vi "MeasLeakRate01.vi"() -> ()   [LabVIEW 2011]
panel:
  out "leak rate (torr/min)":dbl
  out "S20":dbl
  out "S11":dbl
  out "S10":dbl
  out "S01":dbl
  out "S00":dbl
  out "A11":dbl[](array[numeric])
  out "P":dbl
  in  "first":bool=TRUE
  out "A20":dbl[](array[numeric])
  out "A10":dbl[](array[numeric])
  out "A01":dbl[](array[numeric])
  out "A00":dbl[](array[numeric])
  in  "interval (s)":dbl
  in  "stop":bool
  out "P(Torr)":string
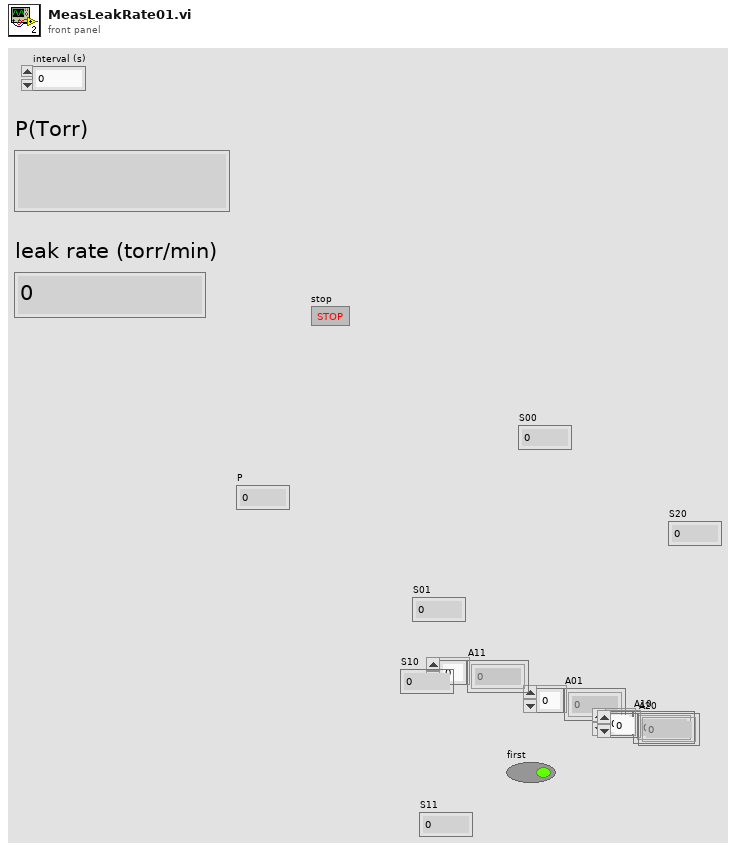
[diagram p1: front panel]
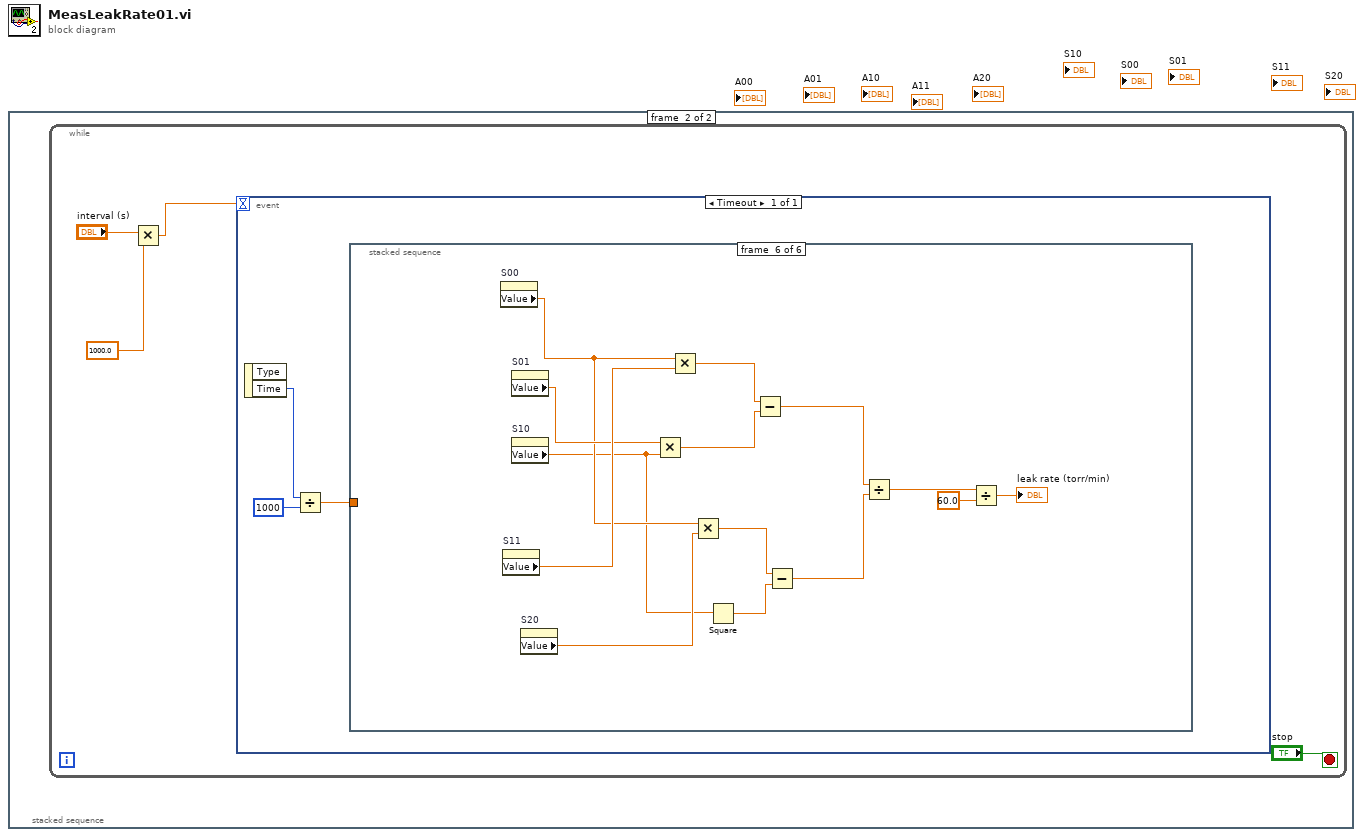
[diagram p0: block diagram]
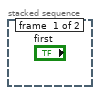
[diagram p2: hidden frame]
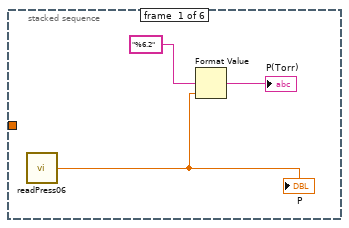
[diagram p3: hidden frame]
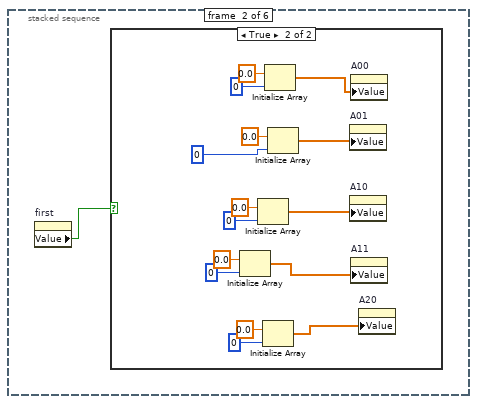
[diagram p4: hidden frame]
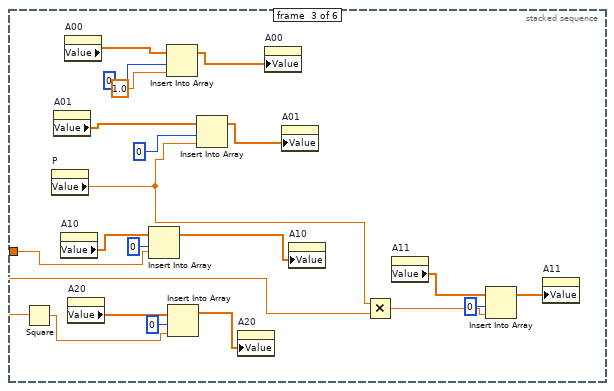
[diagram p6: hidden frame]
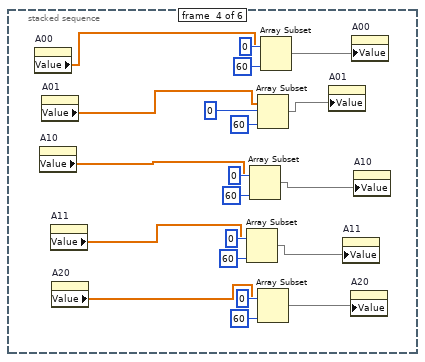
[diagram p7: hidden frame]
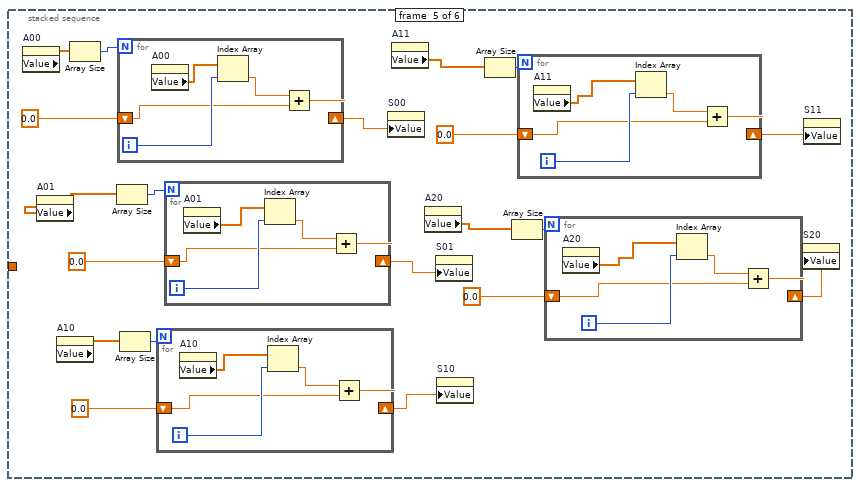
[diagram p8: hidden frame]
diagram:
  n1 = stacked-sequence {
    frame #0 {
    }
    frame #1 {
      n2 = while {
        stop <- "stop" stop-if-true
        n3 = Multiply(x="interval (s)", y=1000.0) -> (x*y=w2:dbl)
        n4 = event shown="[0] Timeout" {
          selector: _ -> [_]
          dyn-events: _ -> [_]
          timeout: w2 -> [_]
          event Timeout {
            n5 = event-data() -> ("Time"=w7:u32)  [unwired: 1 in, 1 out]
            n6 = Divide(x=w7, y=u32 1000) -> (x/y=w5:dbl)
            n7 = stacked-sequence {
              tunnel: w5 -> [_ _ w36 _ _ _]
              frame #0 {
                n8 = call "readPress06.vi"() -> ("P"=w9:dbl)
                "P" <- w9
                n9 = Format Value(format string="%6.2", value (0)=w9) -> (output string=→"P(Torr)":string)  [unwired: 1 in]
              }
              frame #1 {
                n10 = property on="first" class="Bool (strict)"() -> ("Value"=w11:bool)  [unwired: 2 in, 2 out]
                n11 = case shown="True" w11 {
                  frame False {
                  }
                  frame True {
                    n12 = Initialize Array(0.0 ("element"), 0 ("dimension size")) -> (w14:dbl[])
                    n13 = Initialize Array(0.0 ("element"), 0 ("dimension size")) -> (w15:dbl[])
                    n14 = Initialize Array(0.0 ("element"), 0 ("dimension size")) -> (w13:dbl[])
                    n15 = Initialize Array(0.0 ("element"), 0 ("dimension size")) -> (w12:dbl[])
                    n16 = Initialize Array(0.0 ("element"), 0 ("dimension size")) -> (w16:dbl[])
                    n17 = property on="A01" class="Arr (strict)"("Value"=w16) -> ()  [unwired: 2 in, 2 out]
                    n18 = property on="A10" class="Arr (strict)"("Value"=w15) -> ()  [unwired: 2 in, 2 out]
                    n19 = property on="A00" class="Arr (strict)"("Value"=w12) -> ()  [unwired: 2 in, 2 out]
                    n20 = property on="A11" class="Arr (strict)"("Value"=w14) -> ()  [unwired: 2 in, 2 out]
                    n21 = property on="A20" class="Arr (strict)"("Value"=w13) -> ()  [unwired: 2 in, 2 out]
                  }
                }
              }
              frame #2 {
                n22 = Square(x=w36) -> (x^2=w37:dbl)
                n23 = property on="P" class="DigNum (strict)"() -> ("Value"=w35:dbl)  [unwired: 2 in, 2 out]
                n24 = property on="A01" class="Arr (strict)"() -> ("Value"=w42:dbl[])  [unwired: 2 in, 2 out]
                n25 = property on="A10" class="Arr (strict)"() -> ("Value"=w41:dbl[])  [unwired: 2 in, 2 out]
                n26 = property on="A00" class="Arr (strict)"() -> ("Value"=w44:dbl[])  [unwired: 2 in, 2 out]
                n27 = property on="A20" class="Arr (strict)"() -> ("Value"=w39:dbl[])  [unwired: 2 in, 2 out]
                n28 = Insert Into Array(array=w41, index=0, new element=w36) -> (w29:dbl[])
                n29 = Insert Into Array(array=w44, index=0, new element=1.0 ("new element/subarray")) -> (w31:dbl[])
                n30 = Insert Into Array(array=w39, index=0, new element=w37) -> (w30:dbl[])
                n31 = Insert Into Array(array=w42, index=0, new element=w35) -> (w27:dbl[])
                n32 = property on="A20" class="Arr (strict)"("Value"=w30) -> ()  [unwired: 2 in, 2 out]
                n33 = property on="A00" class="Arr (strict)"("Value"=w31) -> ()  [unwired: 2 in, 2 out]
                n34 = property on="A01" class="Arr (strict)"("Value"=w27) -> ()  [unwired: 2 in, 2 out]
                n35 = property on="A10" class="Arr (strict)"("Value"=w29) -> ()  [unwired: 2 in, 2 out]
                n36 = Multiply(x=w35, y=w36) -> (x*y=w33:dbl)
                n37 = property on="A11" class="Arr (strict)"() -> ("Value"=w34:dbl[])  [unwired: 2 in, 2 out]
                n38 = Insert Into Array(array=w34, index=0, new element=w33) -> (w28:dbl[])
                n39 = property on="A11" class="Arr (strict)"("Value"=w28) -> ()  [unwired: 2 in, 2 out]
              }
              frame #3 {
                n40 = property on="A00" class="Arr (strict)"() -> ("Value"=w61:dbl[])  [unwired: 2 in, 2 out]
                n41 = property on="A10" class="Arr (strict)"() -> ("Value"=w52:dbl[])  [unwired: 2 in, 2 out]
                n42 = property on="A01" class="Arr (strict)"() -> ("Value"=w53:dbl[])  [unwired: 2 in, 2 out]
                n43 = property on="A11" class="Arr (strict)"() -> ("Value"=w51:dbl[])  [unwired: 2 in, 2 out]
                n44 = property on="A20" class="Arr (strict)"() -> ("Value"=w64:dbl[])  [unwired: 2 in, 2 out]
                n45 = Array Subset(array=w51, index=0, length=60) -> (w48:dbl[])
                n46 = Array Subset(array=w52, index=0, length=60) -> (w49:dbl[])
                n47 = Array Subset(array=w53, index=0, length=60) -> (w50:dbl[])
                n48 = Array Subset(array=w64, index=0, length=60) -> (w47:dbl[])
                n49 = Array Subset(array=w61, index=0, length=60) -> (w60:dbl[])
                n50 = property on="A01" class="Arr (strict)"("Value"=w50) -> ()  [unwired: 2 in, 2 out]
                n51 = property on="A11" class="Arr (strict)"("Value"=w48) -> ()  [unwired: 2 in, 2 out]
                n52 = property on="A20" class="Arr (strict)"("Value"=w47) -> ()  [unwired: 2 in, 2 out]
                n53 = property on="A00" class="Arr (strict)"("Value"=w60) -> ()  [unwired: 2 in, 2 out]
                n54 = property on="A10" class="Arr (strict)"("Value"=w49) -> ()  [unwired: 2 in, 2 out]
              }
              frame #4 {
                n55 = property on="A00" class="Arr (strict)"() -> ("Value"=w85:dbl[])  [unwired: 2 in, 2 out]
                n56 = property on="A01" class="Arr (strict)"() -> ("Value"=w81:dbl[])  [unwired: 2 in, 2 out]
                n57 = property on="A10" class="Arr (strict)"() -> ("Value"=w78:dbl[])  [unwired: 2 in, 2 out]
                n58 = Array Size(array=w85) -> (size(s)=w86:i32)
                n59 = Array Size(array=w81) -> (size(s)=w83:i32)
                n60 = for {
                  N: w86 -> [_]
                  shift-right: [w107] -> w71
                  shift-left: 0.0 -> [w108]
                  i -> [w110]
                  n61 = property on="A00" class="Arr (strict)"() -> ("Value"=w111:dbl[])  [unwired: 2 in, 2 out]
                  n62 = Index Array(array=w111, index=w110) -> (element=w109:dbl)
                  n63 = Add(x=w109, y=w108) -> (x+y=w107:dbl)
                }
                n64 = Array Size(array=w78) -> (size(s)=w80:i32)
                n65 = for {
                  N: w80 -> [_]
                  shift-right: [w98] -> w70
                  shift-left: 0.0 -> [w99]
                  i -> [w101]
                  n66 = property on="A10" class="Arr (strict)"() -> ("Value"=w97:dbl[])  [unwired: 2 in, 2 out]
                  n67 = Index Array(array=w97, index=w101) -> (element=w100:dbl)
                  n68 = Add(x=w100, y=w99) -> (x+y=w98:dbl)
                }
                n69 = for {
                  N: w83 -> [_]
                  shift-right: [w103] -> w69
                  shift-left: 0.0 -> [w104]
                  i -> [w106]
                  n70 = property on="A01" class="Arr (strict)"() -> ("Value"=w102:dbl[])  [unwired: 2 in, 2 out]
                  n71 = Index Array(array=w102, index=w106) -> (element=w105:dbl)
                  n72 = Add(x=w105, y=w104) -> (x+y=w103:dbl)
                }
                n73 = property on="S00" class="DigNum (strict)"("Value"=w71) -> ()  [unwired: 2 in, 2 out]
                n74 = property on="A11" class="Arr (strict)"() -> ("Value"=w75:dbl[])  [unwired: 2 in, 2 out]
                n75 = property on="A20" class="Arr (strict)"() -> ("Value"=w72:dbl[])  [unwired: 2 in, 2 out]
                n76 = property on="S01" class="DigNum (strict)"("Value"=w69) -> ()  [unwired: 2 in, 2 out]
                n77 = property on="S10" class="DigNum (strict)"("Value"=w70) -> ()  [unwired: 2 in, 2 out]
                n78 = Array Size(array=w75) -> (size(s)=w77:i32)
                n79 = Array Size(array=w72) -> (size(s)=w74:i32)
                n80 = for {
                  N: w77 -> [_]
                  shift-right: [w93] -> w68
                  shift-left: 0.0 -> [w94]
                  i -> [w96]
                  n81 = property on="A11" class="Arr (strict)"() -> ("Value"=w92:dbl[])  [unwired: 2 in, 2 out]
                  n82 = Index Array(array=w92, index=w96) -> (element=w95:dbl)
                  n83 = Add(x=w95, y=w94) -> (x+y=w93:dbl)
                }
                n84 = for {
                  N: w74 -> [_]
                  shift-right: [w88] -> w67
                  shift-left: 0.0 -> [w89]
                  i -> [w91]
                  n85 = property on="A20" class="Arr (strict)"() -> ("Value"=w87:dbl[])  [unwired: 2 in, 2 out]
                  n86 = Index Array(array=w87, index=w91) -> (element=w90:dbl)
                  n87 = Add(x=w90, y=w89) -> (x+y=w88:dbl)
                }
                n88 = property on="S20" class="DigNum (strict)"("Value"=w67) -> ()  [unwired: 2 in, 2 out]
                n89 = property on="S11" class="DigNum (strict)"("Value"=w68) -> ()  [unwired: 2 in, 2 out]
              }
              frame #5 {
                n90 = property on="S00" class="DigNum (strict)"() -> ("Value"=w121:dbl)  [unwired: 2 in, 2 out]
                n91 = property on="S11" class="DigNum (strict)"() -> ("Value"=w125:dbl)  [unwired: 2 in, 2 out]
                n92 = property on="S01" class="DigNum (strict)"() -> ("Value"=w124:dbl)  [unwired: 2 in, 2 out]
                n93 = property on="S10" class="DigNum (strict)"() -> ("Value"=w119:dbl)  [unwired: 2 in, 2 out]
                n94 = property on="S20" class="DigNum (strict)"() -> ("Value"=w120:dbl)  [unwired: 2 in, 2 out]
                n95 = Multiply(x=w124, y=w119) -> (x*y=w122:dbl)
                n96 = Multiply(x=w121, y=w125) -> (x*y=w123:dbl)
                n97 = Multiply(x=w121, y=w120) -> (x*y=w118:dbl)
                n98 = Square(x=w119) -> (x^2=w117:dbl)
                n99 = Subtract(x=w123, y=w122) -> (x-y=w116:dbl)
                n100 = Subtract(x=w118, y=w117) -> (x-y=w115:dbl)
                n101 = Divide(x=w116, y=w115) -> (x/y=w114:dbl)
                n102 = Divide(x=w114, y=60.0) -> (x/y=→"leak rate (torr/min)":dbl)
              }
            }
          }
        }
      }
    }
  }
